vi "上移动.vi"(3 "移动前":u16[][](array[numeric])=[[0, 0, 6, 1], [0, 0, 2, 0], [0, 0, 0, 0], [0, 0, 0, 1]]) -> (0 "移动后":i32[][](array[numeric]), 1 "分数":ext)   [LabVIEW 2013]
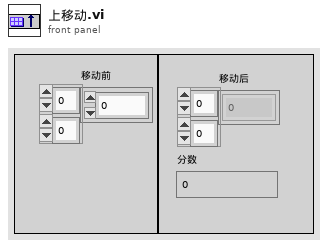
[diagram p1: front panel]
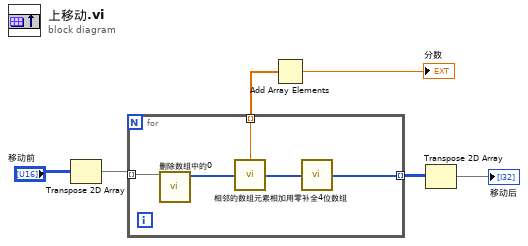
[diagram p0: block diagram]
diagram:
  n1 = Transpose 2D Array(2D array="移动前") -> (transposed array=w5:u16[][])
  n2 = for {
    tunnel: w5 -> [w11] mode=indexing
    tunnel: [w10] -> w4 mode=indexing
    tunnel: [w7] -> w2 mode=indexing
    n3 = call "删除数组中的0.vi"("数组输入"=w11) -> ("数组输出"=w8:u16[])  [unwired: 10 in]
    n4 = call "相邻的数组元素相加.vi"("数组输入"=w8) -> ("数组输出"=w9:i32[], "分数"=w7:ext)  [unwired: 2 in]
    n5 = call "用零补全4位数组.vi"("数组输入"=w9) -> ("数组输出"=w10:i32[])
  }
  n6 = Add Array Elements(numeric array=w2) -> (sum=→"分数":ext)
  n7 = Transpose 2D Array(2D array=w4) -> (transposed array=→"移动后":i32[][])
